vi "Tugas 1.vi"() -> ()   [LabVIEW 2020]
uses:
  <vilib>/MakerHub/LINX/Public/Utilities/Open Serial.vi
  <vilib>/MakerHub/LINX/LMH-LINX.lvlib
  <vilib>/MakerHub/LINX/Public/Sensors/Distance/Ultrasonic/Ultrasonic.lvlib
panel:
  in  "Pin Echo":dbl
  in  "Pin Trigger":dbl
  out "Boolean 3":bool
  out "Boolean 2":bool
  out "Boolean":bool
  in  "Port":refnum<visa-resource-name>
  in  "Stop Button":bool
  out "Tanki Air":dbl(slide) scale=0.0..100.0
  # "Nama : \n1. Aldisya Putra Mahardika\n2. Aurelia Alika Putri Widyanta\n3. Fahmi Fathur Rohman"
  # "MONITORING TANKI AIR"
  # "INDIKATOR"
  # "Keterangan :\nMerah ==> Tanki Air < 20\nOrange => 20 < Tanki Air < 60\nHijau ==> Tank Air > 60"
  # "DATA VALUE"
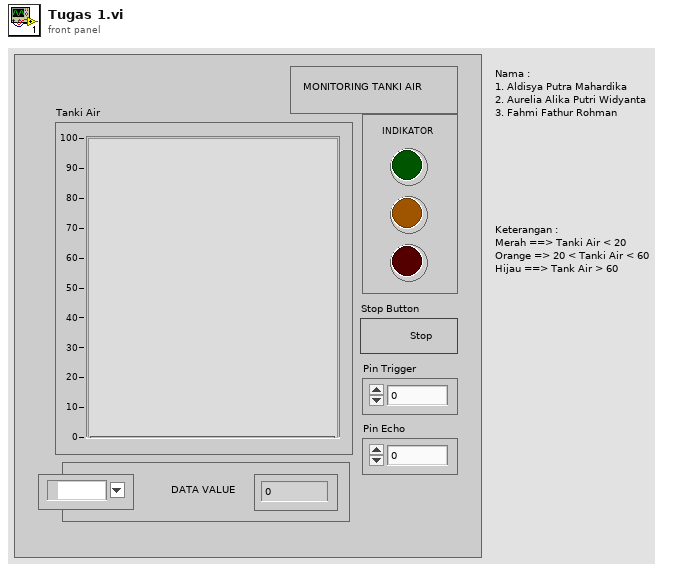
[diagram p1: front panel]
types:
  T1 = typedef "LMH-LINX.lvlib/LINX Ref.ctl" = cluster{"IO":T2, "Interface":T3, "LINX Device Config":T4}
  T2 = typedef "LMH-LINX.lvlib/Platform.ctl" = enum16{"Remote", "Local"}
  T3 = typedef "LMH-LINX.lvlib/Interface.ctl" = enum16{"Serial", "TCP"}
  T4 = typedef "LMH-LINX.lvlib/Device.lvlib/LINX Device Config.ctl" = cluster{"Interface":T3, "COM Port":refnum<visa-resource-name>, "TCP Configuration":T5, "Device Family":u8, "Device ID":u8, "Device Name":string, "TCP Ref":refnum<k5>, "Channels":T6}
  T5 = typedef "LMH-LINX.lvlib/Device.lvlib/TCP Config.ctl" = cluster{"IP Address":string, "Port":u16}
  T6 = typedef "LMH-LINX.lvlib/Channels.ctl" = cluster{"DI":u8[], "DO":u8[], "AI":u8[], "AO":u8[], "PWM":u8[], "QE":u8[], "UART":u8[], "I2C 2":u8[], "SPI":u8[], "CAN":u8[], "Servo":u8[], "AI Ref (V)":dbl, "AI Resolution (Bits)":u8, "AO Ref (V)":dbl, "AO Resolution (Bits)":u8}
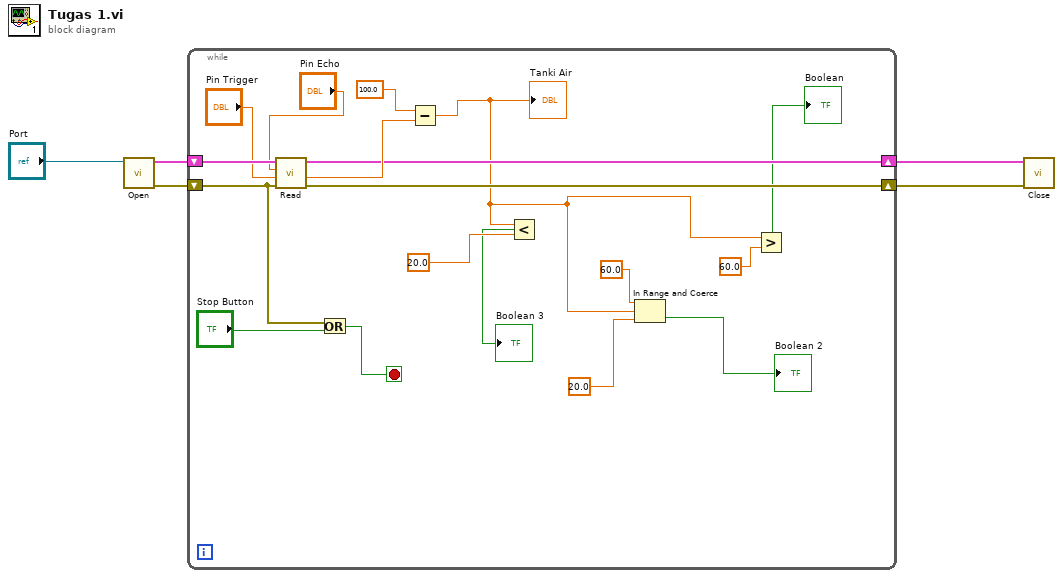
[diagram p0: block diagram]
diagram:
  n1 = call-poly <vilib>:"Open.vi"("Serial Port"="Port") -> ("Error Out"=w3:errorcluster, "LINX Resource"=w5:T1)  [unwired: 8 in, 1 out]
  n2 = while {
    shift-right: [w16] -> w4
    shift-left: w5 -> [w23]
    shift-right: [w15] -> w2
    shift-left: w3 -> [w20]
    stop <- w22 stop-if-true
    n3 = call <vilib>:"Read.vi"("Error In"=w20, "DO Channel"="Pin Trigger", "DI Channel"="Pin Echo", "LINX Resource"=w23) -> ("Error Out"=w15:errorcluster, "Centimeters"=w17:dbl, "LINX Resource"=w16:T1)  [unwired: 4 in, 1 out]
    n4 = Or(x=w20, y="Stop Button") -> (x .or. y?=w22:bool)
    n5 = Subtract(x=100.0, y=w17) -> (x-y=w6:dbl)
    "Tanki Air" <- w6
    n6 = Less?(x=w6, y=20.0) -> (x < y?=→"Boolean 3":bool)
    n7 = In Range and Coerce(upper limit=60.0, x=w6, lower limit=20.0) -> (In Range?=→"Boolean 2":bool)  [unwired: 1 out]
    n8 = Greater?(x=w6, y=60.0) -> (0:→"Boolean":bool)
  }
  n9 = call <vilib>:"Close.vi"("Error In"=w2, "LINX Resource"=w4) -> ()  [unwired: 9 in, 1 out]
